vi "Parse Text-{} UnescapedVariable-Text.vi"(8 "Error In":errorcluster) -> (0 "Error Out":errorcluster)   [LabVIEW 2018, in "Tests.lvlib" / "Parser.lvlib"]
uses:
  Parser.lvlib
  src/Toolkit/Tokens/Text/Text.lvclass
  src/Toolkit/Tokens/UnescapedVariable/UnescapedVariable.lvclass
  src/Toolkit/Tokens/Keyable/API/Keyable.lvclass/Keyable.ctl
  src/Toolkit/Tokens/Keyable/API/Read Key.vi
  src/Toolkit/Readers/String/String.lvclass
  D:/Users/cfield/Code/Field R&D Services/Mustache/trunk/src/Toolkit/Readers/Abstract/Abstract.lvclass
  <vilib>/Utility/LVClass/Get LV Class Name.vi
  src/Toolkit/Tokens/Text/API/Read Content.vi
  <vilib>/addons/_JKI Toolkits/Caraya/classes/Assert/Assert Equal_Variant.vi
  src/Toolkit/Tokens/Keyable/API/Keyable.lvclass
  <vilib>/addons/_JKI Toolkits/Caraya/classes/Test/Test.lvclass
  <vilib>/addons/_JKI Toolkits/Caraya/classes/Assert/Assert.lvclass
  src/Toolkit/Tokens/Abstract/Abstract.lvclass
  Tests.lvlib
  src/Toolkit/Toolkit.lvlib
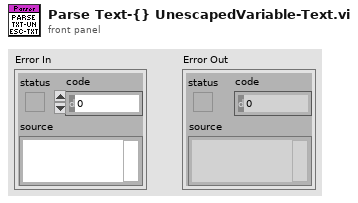
[diagram p1: front panel]
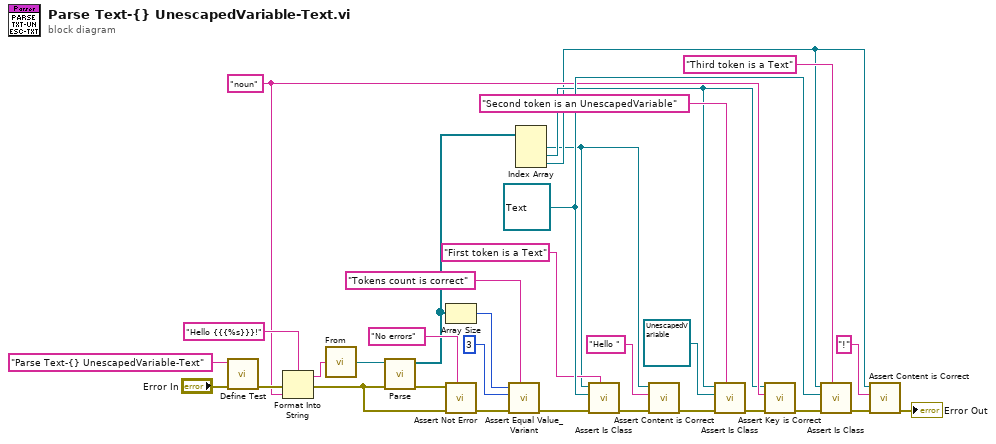
[diagram p0: block diagram]
diagram:
  w13 = refnum<class "Text.lvclass"> refnum ("Mustache.lvlib:Tokens.lvlib:Text.lvclass")
  w9 = "noun" ("String")
  n1 = call <vilib>:"Define Test.vi"("error in (no error)"="Error In", "Label (VI Title)"="Parse Text-{} UnescapedVariable-Text") -> ("error out"=w29:errorcluster)  [unwired: 9 in]
  n2 = Format Into String(format string="Hello {{{%s}}}!", error in=w29, w9) -> (resulting string=w20:string, error out=w2:errorcluster)  [unwired: 1 in]
  n3 = call "From.vi"("String"=w20) -> ("String"=w1:refnum<class "String.lvclass">)
  n4 = call "Parse.vi"("Error In"=w2, "Reader"=w1) -> ("Error Out"=w30:errorcluster, "Tokens"=w22:refnum<class "Abstract.lvclass">[])  [unwired: 8 in]
  n5 = Array Size(array=w22) -> (size(s)=w25:i32)
  n6 = call <vilib>:"Assert Not Error.vi"("Label"="No errors", "error in (no error)"=w2, "Not Error?"=w30) -> ("error out"=w27:errorcluster)  [unwired: 8 in]
  n7 = call <vilib>:"Assert Equal Value_Variant.vi"("Label"="Tokens count is correct", "error in (no error)"=w27, "Y"=3 ("size(s)"), "X"=w25) -> ("error out"=w23:errorcluster)  [unwired: 7 in]
  n8 = Index Array(array=w22) -> (element #1=w3:refnum<class "Abstract.lvclass">, element #2=w7:refnum<class "Abstract.lvclass">, element #3=w5:refnum<class "Abstract.lvclass">)  [unwired: 3 in]
  n9 = call "Assert Is Class.vi"("Label"="First token is a Text", "Error In"=w23, "Expected"=w13, "Actual"=w3) -> ("Error Out"=w19:errorcluster)  [unwired: 7 in]
  n10 = call "Assert Content is Correct.vi"("Error In"=w19, "Expected"="Hello ", "Token"=w3) -> ("Error Out"=w18:errorcluster)  [unwired: 8 in]
  n11 = call "Assert Is Class.vi"("Label"="Second token is an UnescapedVariable", "Error In"=w18, "Expected"=refnum<class "UnescapedVariable.lvclass"> refnum ("Mustache.lvlib:Tokens.lvlib:UnescapedVariable.lvclass"), "Actual"=w7) -> ("Error Out"=w8:errorcluster)  [unwired: 7 in]
  n12 = call "Assert Key is Correct.vi"("Error In"=w8, "Expected"=w9, "Token"=w7) -> ("Error Out"=w17:errorcluster)  [unwired: 8 in]
  n13 = call "Assert Is Class.vi"("Label"="Third token is a Text", "Error In"=w17, "Expected"=w13, "Actual"=w5) -> ("Error Out"=w16:errorcluster)  [unwired: 7 in]
  n14 = call "Assert Content is Correct.vi"("Error In"=w16, "Expected"="!", "Token"=w5) -> ("Error Out"=→"Error Out":errorcluster)  [unwired: 8 in]
